vi "Untitled 7.vi"() -> ()   [LabVIEW 2021]
uses:
  IBar/IBar.lvclass
panel:
  out "String":string
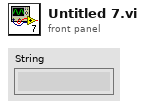
[diagram p1: front panel]
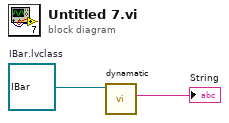
[diagram p0: block diagram]
diagram:
  w2 = refnum<class "IBar.lvclass"> refnum  # IBar.lvclass
  n1 = call-dynamic "dynamatic.vi"("IBar in"=w2) -> ("String"=→"String":string)  [unwired: 8 in, 2 out]
